vi "GetPlotParameter.vi"(8 "error in (no error)":errorcluster caption="错误输入（无错误）", 11 "XYPlot 输入":refnum<class "TrendPlot.lvclass">) -> (0 "error out":errorcluster caption="错误输出", 1 "采样点数":i32, 2 "时间轴":bool, 3 "XYPlot 输出":refnum<class "TrendPlot.lvclass">)   [LabVIEW 2018, in "DataDisplay.lvlib" / "TrendPlot.lvclass"]
uses:
  TrendPlot.lvclass
  TrendPlot.lvclass/TrendPlot.ctl
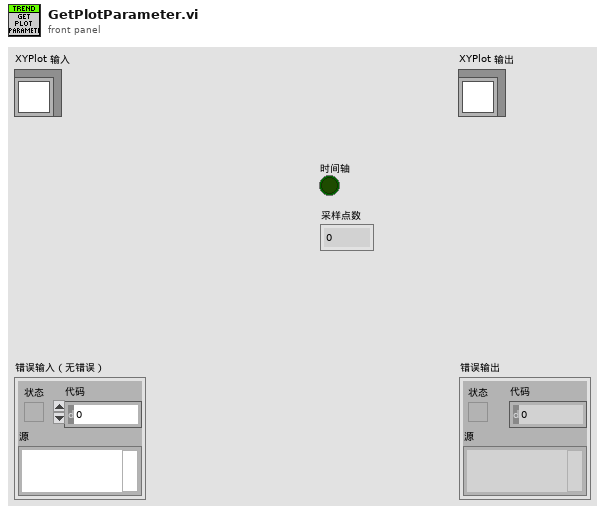
[diagram p1: front panel]
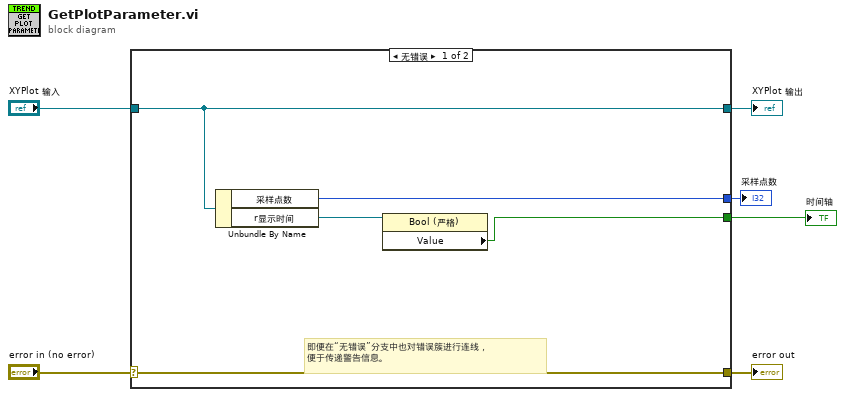
[diagram p0: block diagram]
diagram:
  n1 = case shown="无错误" "error in (no error)" {
    selector: "error in (no error)" -> [w11 w13]
    tunnel: [w11 w13] -> w5
    tunnel: [w10 w12] -> w3
    tunnel: "XYPlot 输入" -> [w10 w12]
    tunnel: [w9 _] -> w2
    tunnel: [w7 _] -> w1
    frame No Error {
      # "即便在“无错误”分支中也对错误簇进行连线，\n便于传递警告信息。"
      n2 = Unbundle By Name(w10) -> ("采样点数"=w9:i32, "r显示时间"=w8:refnum<vi>)
      n3 = property class="Bool (严格)"(reference=w8) -> ("Value"=w7:bool)  [unwired: 1 in, 2 out]
    }
    frame Error {
    }
  }
  "error out" <- w5
  "XYPlot 输出" <- w3
  "采样点数" <- w2
  "时间轴" <- w1
